vi "Save_Data.vi"(8 "error in (no error)":errorcluster, 11 "Array":dbl[][](array[numeric])) -> (0 "error out":errorcluster, 2 "Boolean":bool, 3 "Path":path)   [LabVIEW 2018]
doc: "It saves the file!\n\nInputs:\nArray;\nError In.\n\nOutputs:\nSave File to;\nError Out."
uses:
  <vilib>/Utility/file.llb/Write Delimited Spreadsheet (string).vi
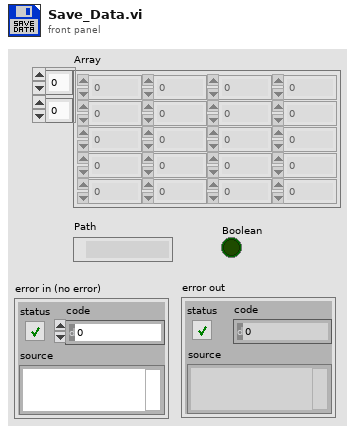
[diagram p1: front panel]
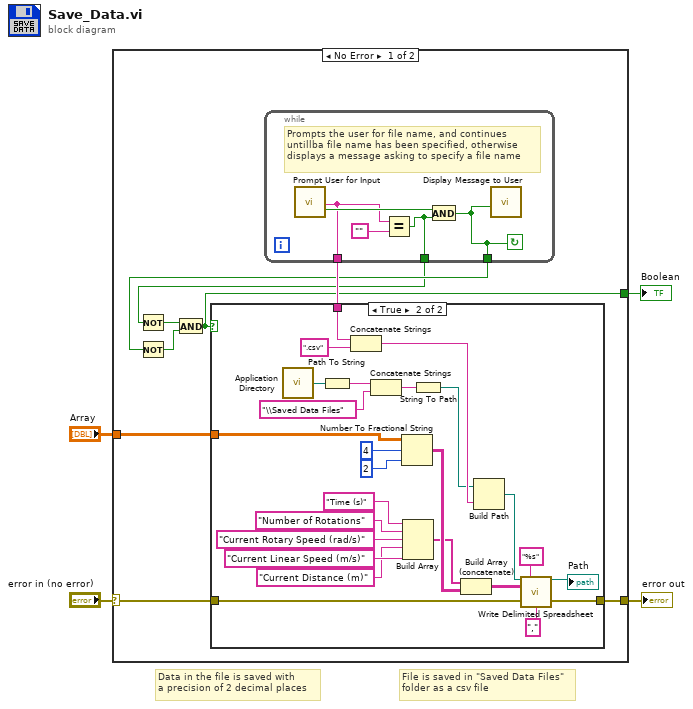
[diagram p0: block diagram]
diagram:
  # "File is saved in \"Saved Data Files\"\nfolder as a csv file"
  # "Data in the file is saved with \na precision of 2 decimal places"
  n1 = case shown="No Error" "error in (no error)" {
    selector: "error in (no error)" -> [w12 w45]
    tunnel: "Array" -> [w13 _]
    tunnel: [w11 w45] -> w3
    tunnel: [w5 _] -> w1
    frame No Error {
      n2 = while {
        tunnel: [w43] -> w10
        tunnel: [w41] -> w9
        tunnel: [w40] -> w8
        stop <- w41 continue-if-true
        # "Prompts the user for file name, and continues\nuntillba file name has been specified, otherwise\ndisplays a message asking to specify a file name"
        n3 = call "Prompt User for Input"() -> ("File Name"=w43:string, "OK"=w44:bool)  [unwired: 17 in, 1 out]
        n4 = Equal?(x=w43, y="") -> (x = y?=w40:bool)
        n5 = And(x=w44, y=w40) -> (x .and. y?=w41:bool)
        n6 = call "Display Message to User"("Enable"=w41) -> ()  [unwired: 9 in, 2 out]
      }
      n7 = Not(x=w8) -> (.not. x?=w6:bool)
      n8 = Not(x=w9) -> (.not. x?=w7:bool)
      n9 = And(x=w6, y=w7) -> (x .and. y?=w5:bool)
      n10 = case shown="True" w5 {
        tunnel: w13 -> [_ w32]
        tunnel: w12 -> [w14 w31]
        tunnel: [w14 w30] -> w11
        tunnel: w10 -> [_ w23]
        frame False {
        }
        frame True {
          n11 = call <vilib>:"Application Directory.vi"() -> ("Application Directory"=w18:path)
          n12 = Path To String(path=w18) -> (string=w17:string)
          n13 = Concatenate Strings(w23, ".csv" ("name or relative path")) -> (w21:string)
          n14 = Concatenate Strings(w17, "\\Saved Data Files") -> (w16:string)
          n15 = Number To Fractional String(number=w32, width (-)=i16 4, precision (6)=i16 2) -> (F-format string=w33:string[][])  [unwired: 1 in]
          n16 = Build Array("Time (s)", "Number of Rotations", "Current Rotary Speed (rad/s)" ("element"), "Current Distance (m)" ("element"), "Current Linear Speed (m/s)" ("element")) -> (w24:string[])
          n17 = String To Path(string=w16) -> (path=w15:path)
          n18 = Build Array (concatenate)(w24, w33) -> (w34:string[][])
          n19 = Build Path(base path=w15, name or relative path=w21) -> (appended path=w25:path)
          n20 = call-poly <vilib>:"Write Delimited Spreadsheet.vi"("file path (dialog if empty)"=w25, "format (%s)"="%s", "2D data"=w34, "error in (no error)"=w31, "delimiter (\\t)"="," ("delimiter (\\t)")) -> ("new file path (Not A Path if cancelled)"=→"Path":path, "error out"=w30:errorcluster)  [unwired: 9 in]
        }
      }
    }
    frame Error {
    }
  }
  "error out" <- w3
  "Boolean" <- w1
